vi "VariableManager.vi"(7 "Operation":enum16{"Get Tag", "Set Tag"}(ring), 9 "Value":dbl, 11 "Tag":string) -> (1 "Value out":dbl, 3 "Tag Out":string, 4 "Found":bool, 5 "All Tags":cluster{"Tags":string[], "Values":dbl[]})   [LabVIEW 2011]
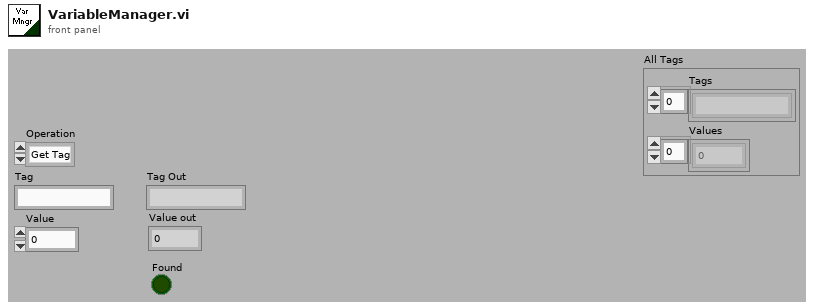
[diagram p1: front panel]
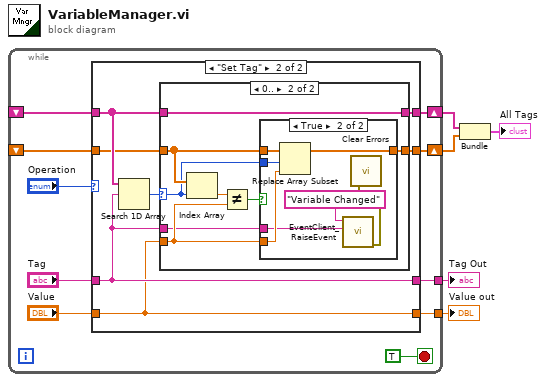
[diagram p0: block diagram]
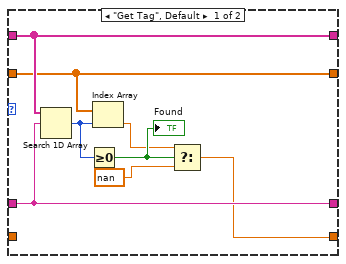
[diagram p2: hidden frame]
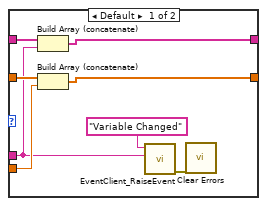
[diagram p3: hidden frame]
diagram:
  n1 = while {
    shift-right: [w14] -> w3
    shift-left: _ -> [w15]
    shift-right: [w12] -> w2
    shift-left: _ -> [w13]
    tunnel: [w8] -> w5
    tunnel: [w7] -> w4
    stop <- TRUE stop-if-true
    n2 = case shown="\"Set Tag\"" "Operation" {
      tunnel: w15 -> [w23 w29]
      tunnel: [w23 w28] -> w14
      tunnel: w13 -> [w22 w26]
      tunnel: [w22 w27] -> w12
      tunnel: "Tag" -> [w21 w25]
      tunnel: "Value" -> [_ w24]
      tunnel: [w21 w25] -> w8
      tunnel: [w17 w24] -> w7
      frame "Get Tag", Default {
        n3 = Search 1D Array(1D array=w23, element=w21) -> (index of element=w20:i32)  [unwired: 1 out]
        n4 = Greater Or Equal To 0?(x=w20) -> (x >= 0?=w19:bool)
        "Found" <- w19
        n5 = Index Array(array=w22, index=w20) -> (element=w18:dbl)
        n6 = Select(t=w18, s=w19, f=nan) -> (s? t:f=w17:dbl)
      }
      frame "Set Tag" {
        n7 = Search 1D Array(1D array=w29, element=w25) -> (index of element=w30:i32)  [unwired: 1 out]
        n8 = case shown="0.." w30 {
          selector: w30 -> [_ w41]
          tunnel: [w37 w46] -> w28
          tunnel: w29 -> [w38 w46]
          tunnel: [w35 w42] -> w27
          tunnel: w26 -> [w36 w43]
          tunnel: w25 -> [w32 w39]
          tunnel: w24 -> [w34 w40]
          frame Default {
            n9 = Build Array (concatenate)(w38, w32) -> (w37:string[])
            n10 = Build Array (concatenate)(w36, w34) -> (w35:dbl[])
            n11 = call "EventClient_RaiseEvent.vi"("Data"=w32, "Event"="Variable Changed") -> ("error out"=w31:errorcluster)  [unwired: 2 in, 7 out]
            n12 = call <vilib>:"Clear Errors.vi"("error in (no error)"=w31) -> ()  [unwired: 7 out]
          }
          frame 0.. {
            n13 = Index Array(array=w43, index=w41) -> (element=w45:dbl)
            n14 = Not Equal?(x=w45, y=w40) -> (x != y?=w44:bool)
            n15 = case shown="True" w44 {
              tunnel: w43 -> [w47 w54]
              tunnel: [w47 w53] -> w42
              tunnel: w41 -> [_ w52]
              tunnel: w40 -> [_ w51]
              tunnel: w39 -> [_ w49]
              frame False {
              }
              frame True {
                n16 = Replace Array Subset(array=w54, new element=w51, index=w52) -> (w53:dbl[])
                n17 = call "EventClient_RaiseEvent.vi"("Data"=w49, "Event"="Variable Changed") -> ("error out"=w48:errorcluster)  [unwired: 2 in, 7 out]
                n18 = call <vilib>:"Clear Errors.vi"("error in (no error)"=w48) -> ()  [unwired: 7 out]
              }
            }
          }
        }
      }
    }
  }
  "Tag Out" <- w5
  "Value out" <- w4
  n19 = Bundle(w3, w2) -> (→"All Tags":cluster{string[], dbl[]})  [unwired: 1 out]
